vi "AlazarForceTrigger.vi"(0 "Handle":u64, 1 "error in (no error)":errorcluster) -> (2 "Handle":u64, 3 "Return Code":u32, 4 "error out":errorcluster)   [LabVIEW 2018]
doc: "Generate a software trigger event."
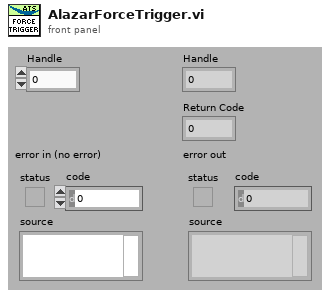
[diagram p1: front panel]
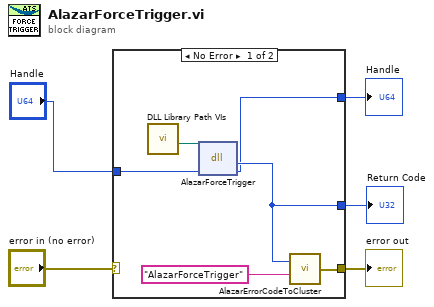
[diagram p0: block diagram]
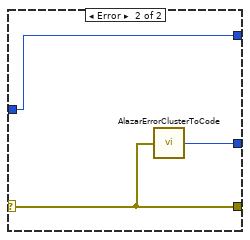
[diagram p2: hidden frame]
diagram:
  n1 = case shown="No Error" "error in (no error)" {
    selector: "error in (no error)" -> [_ w14]
    tunnel: [w8 w14] -> w4
    tunnel: [w10 w13] -> w3
    tunnel: "Handle" -> [w11 w12]
    tunnel: [w7 w12] -> w1
    frame No Error {
      n2 = call "DLL Library Path VIs.vi"() -> ("Alazar"=w6:path)  [unwired: 9 in, 2 out]
      n3 = dll-call lib="C:/Project/SerialSectOCT - FFT GPU/SerialSectOCT/Labview Software/DLL/ATSApi.dll" fn="AlazarForceTrigger"(path in=w6, "handle"=w11) -> ("return type"=w10:u32, "handle"=w7:u64)  [unwired: 2 in, 2 out]
      n4 = call "AlazarErrorCodeToCluster.vi"("Message"="AlazarForceTrigger", "Error Code"=w10) -> ("error out"=w8:errorcluster)
    }
    frame Error {
      n5 = call "AlazarErrorClusterToCode.vi"("error in (no error)"=w14) -> ("Error Code"=w13:u32)
    }
  }
  "Handle" <- w1
  "error out" <- w4
  "Return Code" <- w3
